vi "Message Nested Object.vi"(8 "error in (no error)":errorcluster, 9 "Message":refnum<class "Message.lvclass">, 10 "Name":string, 11 "Application Controller in":refnum<class "Template Module.lvclass">) -> (0 "error out":errorcluster, 3 "Application Controller out":refnum<class "Template Module.lvclass">)   [LabVIEW 2016, in "Template Module.lvclass"]
uses:
  Template Module.lvclass
  <vilib>/ActorFramework/Message/Message.lvclass
  <vilib>/ActorFramework/Message Enqueuer/Message Enqueuer.lvclass/Message Enqueuer.ctl
  <vilib>/ActorFramework/Message Priority Queue/Priority Enqueue.vi
  <vilib>/ActorFramework/Message Enqueuer/Message Enqueuer.lvclass
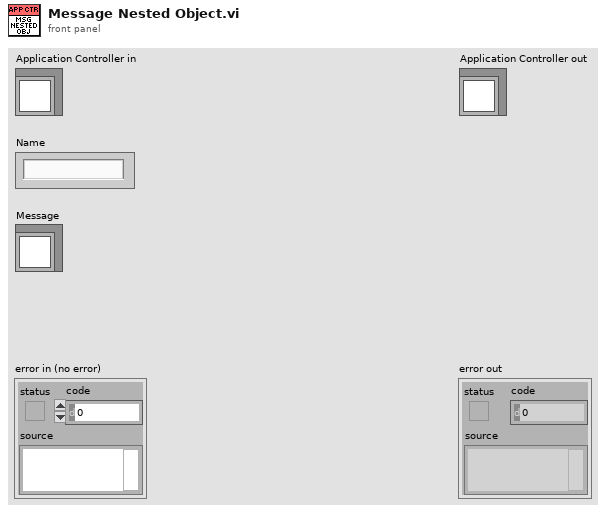
[diagram p1: front panel]
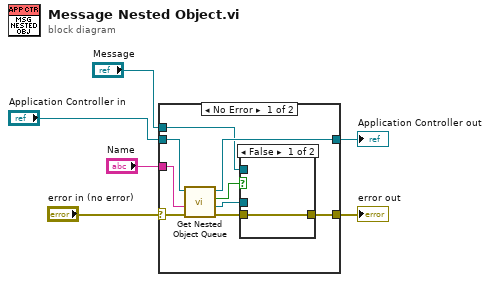
[diagram p0: block diagram]
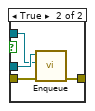
[diagram p2: hidden frame]
diagram:
  n1 = case shown="No Error" "error in (no error)" {
    selector: "error in (no error)" -> [w11 w22]
    tunnel: [w7 w22] -> w5
    tunnel: [w12 w21] -> w3
    tunnel: "Application Controller in" -> [w13 w21]
    tunnel: "Name" -> [w15 _]
    tunnel: "Message" -> [w8 _]
    frame No Error {
      n2 = call-dynamic "Get Nested Object Queue.vi"("error in (no error)"=w11, "Name"=w15, "Measure Object in"=w13) -> ("error out"=w9:errorcluster, "Object Enqueuer"=w10:refnum<class "Message Enqueuer.lvclass">, "Found?"=w14:bool, "Measure Object out"=w12:refnum<class "Template Module.lvclass">)  [unwired: 5 in]
      n3 = case shown="False" w14 {
        tunnel: w10 -> [_ w20]
        tunnel: w9 -> [w16 w19]
        tunnel: w8 -> [_ w18]
        tunnel: [w16 w17] -> w7
        frame False {
        }
        frame True {
          n4 = call <vilib>:"Enqueue.vi"("error in (no error)"=w19, "Message"=w18, "Message Enqueuer in"=w20) -> ("error out"=w17:errorcluster)  [unwired: 7 in, 1 out]
        }
      }
    }
    frame Error {
    }
  }
  "error out" <- w5
  "Application Controller out" <- w3
